vi "MCL Release All Handles.vi"   [LabVIEW 2017, in "Madlib.lvlib"]
doc: "MADLIB_API void MCL_ReleaseAllHandles();"
uses:
  Madlib.lvlib
  Madlib.dll
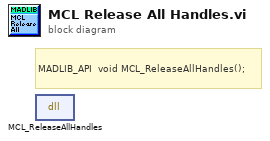
[diagram p0: block diagram]
diagram:
  # "MADLIB_API  void\tMCL_ReleaseAllHandles();"
  n1 = dll-call lib="C:/Users/francesco/dev/pump-probe/Piezo/lvlib/Madlib.*" fn="MCL_ReleaseAllHandles"() -> ()  [unwired: 4 in, 2 out]
